vi "TDM Transfer Simulation.vi"() -> ()   [LabVIEW 2013]
uses:
  <vilib>/rvi/DesktopExecutionNode/Execution/niFpgaDEN_Execute.vi
  <vilib>/rvi/DesktopExecutionNode/DesktopExecutionNode.xnode
  Source/I2S-TDM.lvlib
panel:
  in  "Loop Wait":u32(slide)=45 min=10 max=70 step=1 scale=10.0..70.0
  in  "channel count":u8=2
  in  "transmit":bool
  in  "pause":bool
  in  "24-bit data":bool[](array[boolean])=[TRUE, FALSE, FALSE, TRUE, TRUE, FALSE, FALSE, TRUE, FALSE, TRUE, FALSE, FALSE, FALSE, FALSE, FALSE, FALSE, FALSE, FALSE, FALSE, FALSE, FALSE, FALSE, FALSE, TRUE]
  out "Digital Waveform Graph":digitalwaveform(graph)
  in  "bits per channel":u8=32
  in  "stop":bool
  # "MSB"
  # "LSB"
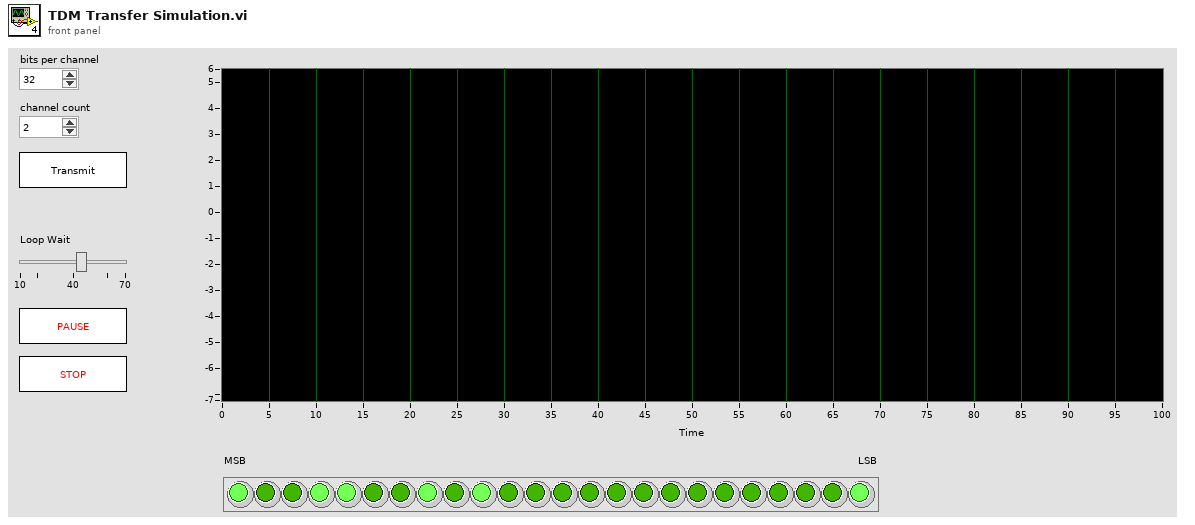
[diagram p1: front panel]
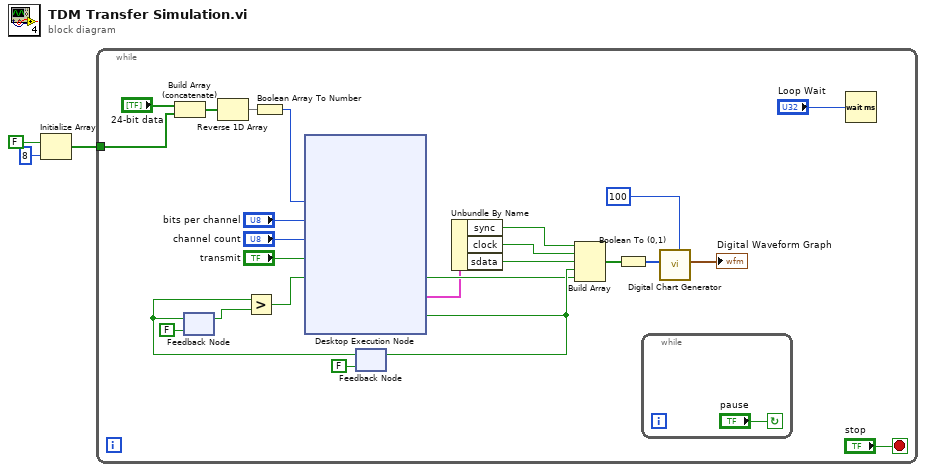
[diagram p0: block diagram]
diagram:
  n1 = Initialize Array(FALSE, 8 ("dimension size")) -> (w1:bool[])
  n2 = while {
    tunnel: w1 -> [w24]
    stop <- "stop" stop-if-true
    n3 = Build Array (concatenate)("24-bit data", w24) -> (w23:bool[])
    n4 = feedback #1(FALSE ("ready for input")) -> (w16:bool)
    n5 = Reverse 1D Array(array=w23) -> (reversed array=w22:bool[])
    n6 = Boolean Array To Number(Boolean array=w22) -> (number=w15:u32)
    n7 = feedback #2(FALSE ("ready for input")) -> (w18:bool)
    n8 = feedback-in #1(w18) -> ()
    n9 = Greater?(x=w18, y=w16) -> (0:w13:bool)
    n10 = xnode "Desktop Execution Node"("sample"=w15, "transfer length"="bits per channel", "channel count"="channel count", "transmit"="transmit", "input valid"=w13) -> ("input valid"=w10:bool, "signals out"=w4:cluster{"clock":bool, "sync":bool, "sdata":bool}, "ready for input"=w11:bool)  [unwired: 1 in, 1 out]
    n11 = feedback-in #2(w11) -> ()
    n12 = Unbundle By Name(w4) -> ("sync"=w7:bool, "clock"=w8:bool, "sdata"=w9:bool)
    n13 = Build Array(w7, w8, w9, w11, w10) -> (w20:bool[])
    n14 = Boolean To (0,1)(Boolean=w20) -> (0, 1=w19:i16[])
    n15 = while {
      stop <- "pause" continue-if-true
    }
    n16 = call "Digital Chart Generator.vi"("History Size"=100, "Input"=w19) -> ("Digital Data"=→"Digital Waveform Graph":digitalwaveform)  [unwired: 9 in]
    n17 = Wait (ms)(milliseconds to wait="Loop Wait") -> ()  [unwired: 1 out]
  }
